vi "Power Read Array.vi"(8 "error in":errorcluster, 11 "Power Supply In":refnum<class "Power Supply.lvclass">) -> (0 "error out":errorcluster, 2 "Power.SP":dbl[](array[numeric]), 3 "Power Supply Out":refnum<class "Power Supply.lvclass">)   [LabVIEW 2023, in "Power Supply.lvclass"]
uses:
  Power Supply.lvclass
  Power Supply.lvclass/Power Supply.ctl
  Low Level Capabilities/Power/Power Setpoint/Power Setpoint.lvclass
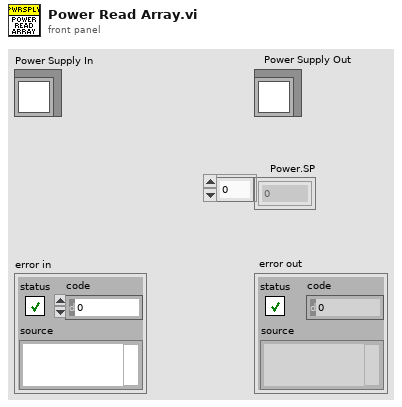
[diagram p1: front panel]
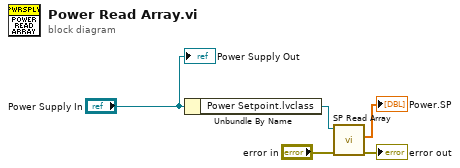
[diagram p0: block diagram]
diagram:
  n1 = Unbundle By Name("Power Supply In") -> ("Power Setpoint.lvclass"=w1:refnum<class "Power Setpoint.lvclass">)
  n2 = call-dynamic "SP Read Array.vi"("error in"="error in", "Power Setpoint in"=w1) -> ("error out"=→"error out":errorcluster, "Current Setpoint"=→"Power.SP":dbl[])  [unwired: 6 in, 2 out]
  "Power Supply Out" <- "Power Supply In"
